vi "Configure Module.vi"(8 "error in (no error)":errorcluster, 10 "IOV ref in":refnum<k21>, 11 "9403 in":refnum<class "9403.lvclass">) -> (0 "error out":errorcluster, 2 "IOV ref out":refnum<k21>, 3 "9403 out":refnum<class "9403.lvclass">)   [LabVIEW 2019, in "Modules.lvlib" / "9403.lvclass"]
uses:
  9403.lvclass
  9403.lvclass/9403.ctl
  <resource>/objmgr/cRIO.rc
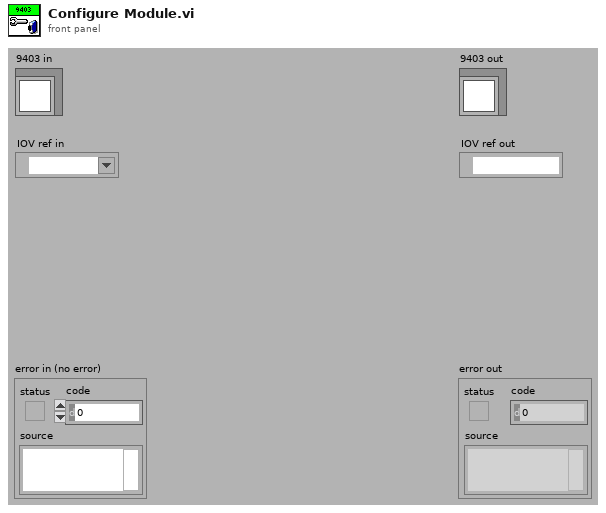
[diagram p1: front panel]
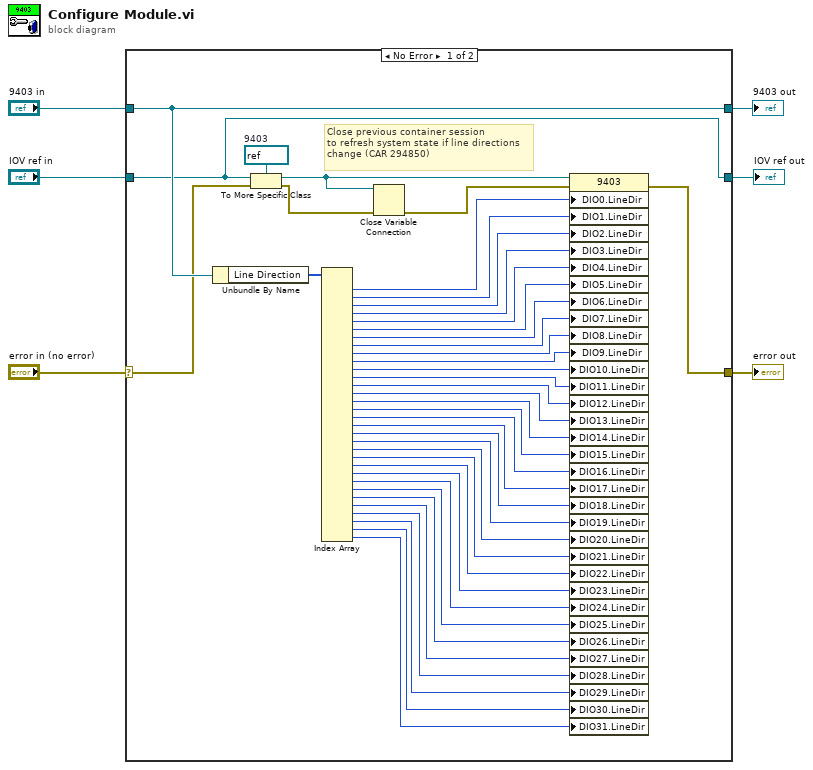
[diagram p0: block diagram]
diagram:
  n1 = case shown="No Error" "error in (no error)" {
    selector: "error in (no error)" -> [w46 w50]
    tunnel: [w44 w50] -> w5
    tunnel: [w47 w49] -> w3
    tunnel: "9403 in" -> [w47 w49]
    tunnel: "IOV ref in" -> [w43 w48]
    tunnel: [w43 w48] -> w1
    frame No Error {
      w45 = refnum<k21> refnum  # 9403
      # "Close previous container session\nto refresh system state if line directions\nchange (CAR 294850)"
      n2 = Unbundle By Name(w47) -> ("Line Direction"=w42:u32[])
      n3 = To More Specific Class(target class=w45, reference=w43, error in=w46) -> (specific class reference=w9:refnum<k21>, error out=w8:errorcluster)
      n4 = Index Array(array=w42) -> (element #1=w41:u32, element #2=w40:u32, element #3=w39:u32, element #4=w38:u32, element #5=w37:u32, element #6=w36:u32, element #7=w35:u32, element #8=w34:u32, element #9=w33:u32, element #10=w32:u32, element #11=w31:u32, element #12=w30:u32, element #13=w29:u32, element #14=w28:u32, element #15=w27:u32, element #16=w26:u32, element #17=w25:u32, element #18=w24:u32, element #19=w23:u32, element #20=w22:u32, element #21=w21:u32, element #22=w20:u32, element #23=w19:u32, element #24=w18:u32, element #25=w17:u32, element #26=w16:u32, element #27=w15:u32, element #28=w14:u32, element #29=w13:u32, element #30=w12:u32, element #31=w11:u32, element #32=w10:u32)  [unwired: 32 in]
      n5 = Close Variable Connection(8:w8, 11:w9) -> (0:w7:errorcluster)
      n6 = property class="9403"(reference=w9, error in=w7, "DIO0.LineDir"=w41, "DIO1.LineDir"=w40, "DIO2.LineDir"=w39, "DIO3.LineDir"=w38, "DIO4.LineDir"=w37, "DIO5.LineDir"=w36, "DIO6.LineDir"=w35, "DIO7.LineDir"=w34, "DIO8.LineDir"=w33, "DIO9.LineDir"=w32, "DIO10.LineDir"=w31, "DIO11.LineDir"=w30, "DIO12.LineDir"=w29, "DIO13.LineDir"=w28, "DIO14.LineDir"=w27, "DIO15.LineDir"=w26, "DIO16.LineDir"=w25, "DIO17.LineDir"=w24, "DIO18.LineDir"=w23, "DIO19.LineDir"=w22, "DIO20.LineDir"=w21, "DIO21.LineDir"=w20, "DIO22.LineDir"=w19, "DIO23.LineDir"=w18, "DIO24.LineDir"=w17, "DIO25.LineDir"=w16, "DIO26.LineDir"=w15, "DIO27.LineDir"=w14, "DIO28.LineDir"=w13, "DIO29.LineDir"=w12, "DIO30.LineDir"=w11, "DIO31.LineDir"=w10) -> (error out=w44:errorcluster)  [unwired: 1 out]
    }
    frame Error {
    }
  }
  "error out" <- w5
  "9403 out" <- w3
  "IOV ref out" <- w1
